vi "TimeoutRole.vi"(8 "error in (no error)":errorcluster, 9 "Game in":refnum<class "Game.lvclass">, 10 "Robot in":refnum<class "Robot.lvclass">, 11 "TimeoutRole in":refnum<class "TimeoutRole.lvclass">) -> (0 "error out":errorcluster, 1 "Game out":refnum<class "Game.lvclass">, 2 "Robot out":refnum<class "Robot.lvclass">, 3 "TimeoutRole out":refnum<class "TimeoutRole.lvclass">)   [LabVIEW 2018, in "TimeoutRole.lvclass"]
uses:
  TimeoutRole.lvclass
  C:/Users/nicolas.oliveira/roboime/SSL_AI/Role_class/Role.lvclass
  Robot_class/Robot.lvclass
  Game_class/Game.lvclass
  Role_class/Role.lvclass/Role.ctl
  Tacticbook_class/Tacticbook.lvclass/Tacticbook.ctl
  Tacticbook_class/Read TimeoutTactic.vi
  TimeoutTactic_class/Read States.vi
  Tacticbook_class/Write TimeoutTactic.vi
  Role_class/Read Tacticbook.vi
  Role_class/Read tactic_index.vi
  Role_class/Write Tacticbook.vi
  Role_class/Write tactic_index.vi
  Tacticbook_class/Tacticbook.lvclass
  TimeoutTactic_class/TimeoutTactic.lvclass
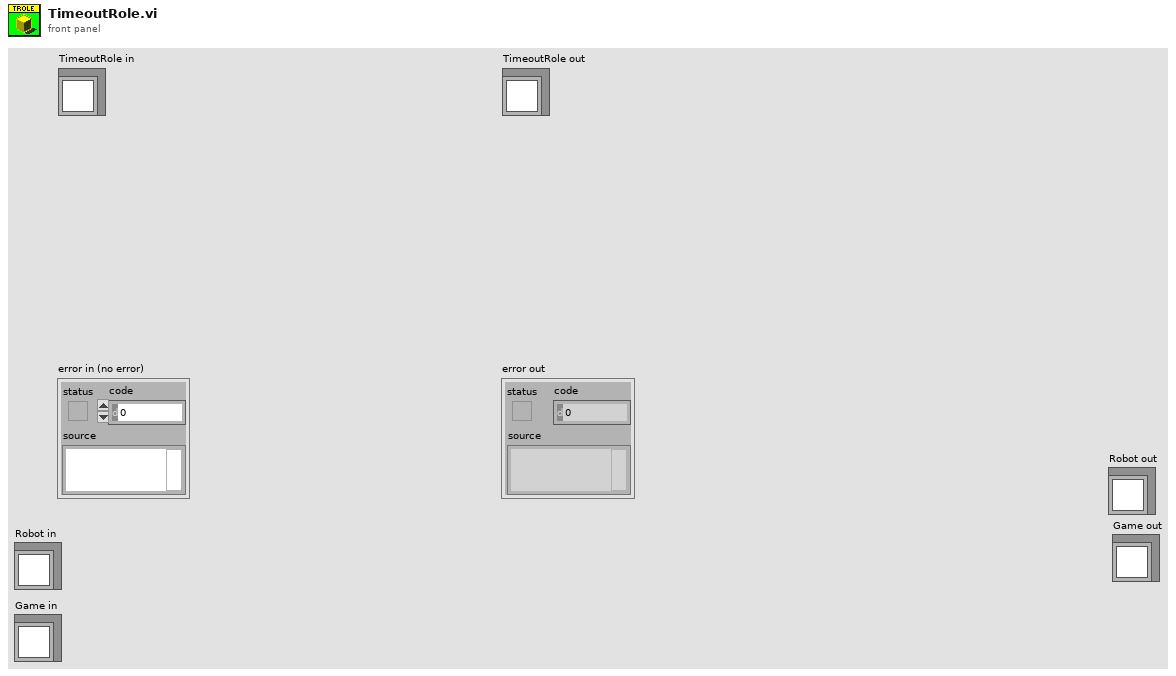
[diagram p1: front panel]
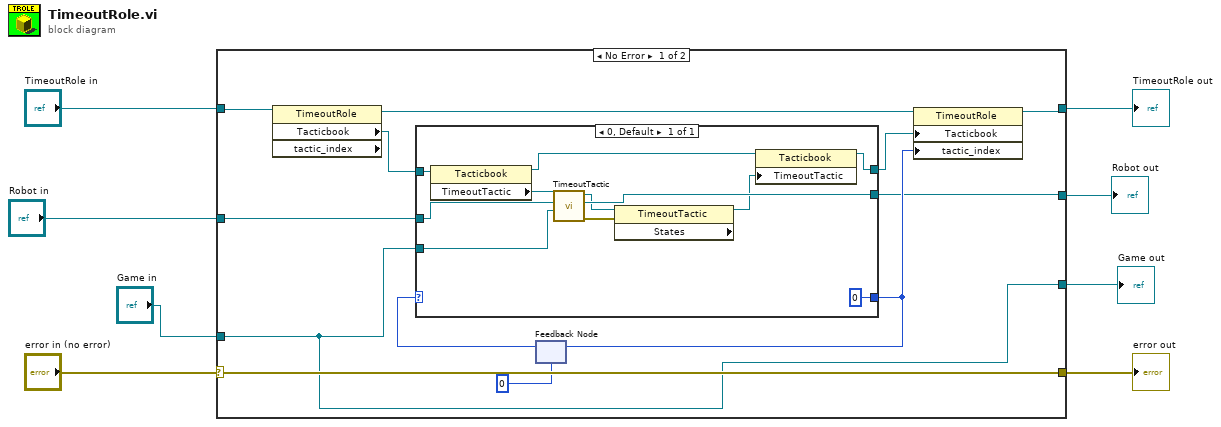
[diagram p0: block diagram]
diagram:
  n1 = case shown="No Error" "error in (no error)" {
    selector: "error in (no error)" -> [w20 w35]
    tunnel: [w20 w35] -> w7
    tunnel: [w9 w34] -> w5
    tunnel: "TimeoutRole in" -> [w13 w34]
    tunnel: "Robot in" -> [w12 w33]
    tunnel: "Game in" -> [w10 w32]
    tunnel: [w11 w33] -> w2
    tunnel: [w10 w32] -> w1
    frame No Error {
      n2 = property class="TimeoutRole" props=["Tacticbook", "tactic_index"](reference=w13) -> (reference out=w19:refnum<class "TimeoutRole.lvclass">, "Tacticbook"=w16:refnum<class "Tacticbook.lvclass">)  [unwired: 1 in, 2 out]
      n3 = feedback #1(0) -> (w17:i32)
      n4 = case shown="0, Default" w17 {
        tunnel: [0] -> w15
        tunnel: w16 -> [w31]
        tunnel: w12 -> [w24]
        tunnel: [w30] -> w11
        tunnel: [w26] -> w14
        tunnel: w10 -> [w22]
        frame 0, Default {
          n5 = property class="Tacticbook"(reference=w31) -> (reference out=w28:refnum<class "Tacticbook.lvclass">, "TimeoutTactic"=w25:refnum<class "TimeoutTactic.lvclass">)  [unwired: 1 in, 1 out]
          n6 = call-dynamic "TimeoutTactic.vi"("Game in"=w22, "Robot"=w24, "TimeoutTactic in"=w25) -> ("error out"=w29:errorcluster, "Robot out"=w30:refnum<class "Robot.lvclass">, "TimeoutTactic out"=w23:refnum<class "TimeoutTactic.lvclass">)  [unwired: 6 in]
          n7 = property class="TimeoutTactic" props=["States"](reference=w23, error in=w29) -> (reference out=w27:refnum<class "TimeoutTactic.lvclass">)  [unwired: 2 out]
          n8 = property class="Tacticbook"(reference=w28, "TimeoutTactic"=w27) -> (reference out=w26:refnum<class "Tacticbook.lvclass">)  [unwired: 1 in, 1 out]
        }
      }
      n9 = feedback-in #1(w15) -> ()
      n10 = property class="TimeoutRole"(reference=w19, "Tacticbook"=w14, "tactic_index"=w15) -> (reference out=w9:refnum<class "TimeoutRole.lvclass">)  [unwired: 1 in, 1 out]
    }
    frame Error {
    }
  }
  "error out" <- w7
  "TimeoutRole out" <- w5
  "Robot out" <- w2
  "Game out" <- w1
